vi "Get Status.vi"(8 "error in (no error)":errorcluster, 11 "Scanner.lvclass in":refnum<class "Scanner.lvclass">) -> (0 "error out":errorcluster, 2 "Status":string, 3 "Scanner.lvclass out":refnum<class "Scanner.lvclass">)   [LabVIEW 2009, in "Scanner.lvclass"]
uses:
  Scanner.lvclass
  Scanner.lvclass/Scanner.ctl
  Instruments/Utility Classes/Scannable/Scannable.lvclass
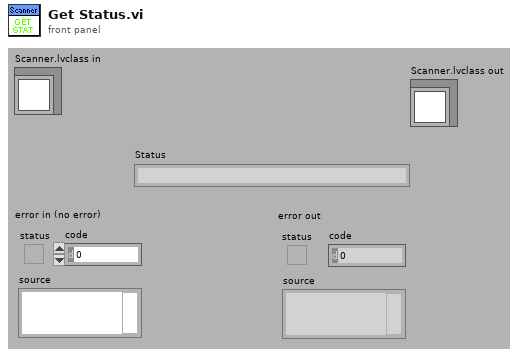
[diagram p1: front panel]
types:
  T1 = typedef "Scanner.lvclass/Range.ctl" = cluster{"xi":dbl, "xf":dbl, "dx":dbl, "Return to...?":bool, "Return to":dbl}
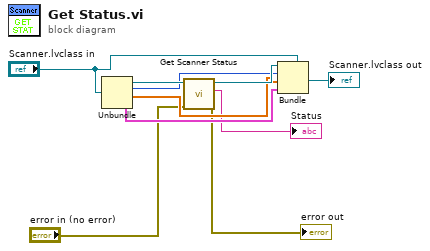
[diagram p0: block diagram]
diagram:
  n1 = Unbundle("Scanner.lvclass in") -> (w10:refnum<class "Scannable.lvclass">, w8:u32, w7:dbl[], w6:T1)
  n2 = call "Get Scanner Status.vi"("error in (no error)"="error in (no error)", "Scannable.lvclass in"=w10) -> ("error out"=→"error out":errorcluster, "Status"=→"Status":string, "Scannable.lvclass out"=w9:refnum<class "Scannable.lvclass">)  [unwired: 7 in]
  n3 = Bundle(cluster="Scanner.lvclass in", w9, w8, w7, w6) -> (→"Scanner.lvclass out":refnum<class "Scanner.lvclass">)
